vi "Example1.vi"() -> ()   [LabVIEW 2019]
uses:
  API/KafkaConsumerEvent.ctl
panel:
  out "size(s)":i32
  out "Events":T1[](array[typedef])
  in  "Topic":string="qamData"
  in  "Partition":i32
  in  "Kafka Broker":string="getafix.ni.corp.natinst.com:9092"
  in  "error in (no error)":errorcluster
  out "error out":errorcluster
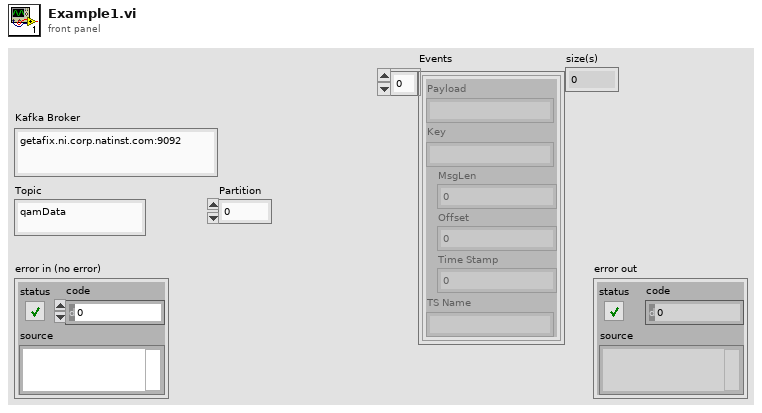
[diagram p1: front panel]
types:
  T1 = typedef "KafkaConsumerEvent.ctl" = cluster{"Payload":string, "Key":string, "MsgLen":u64, "Offset":i64, "Time Stamp":i64, "TS Name":string}
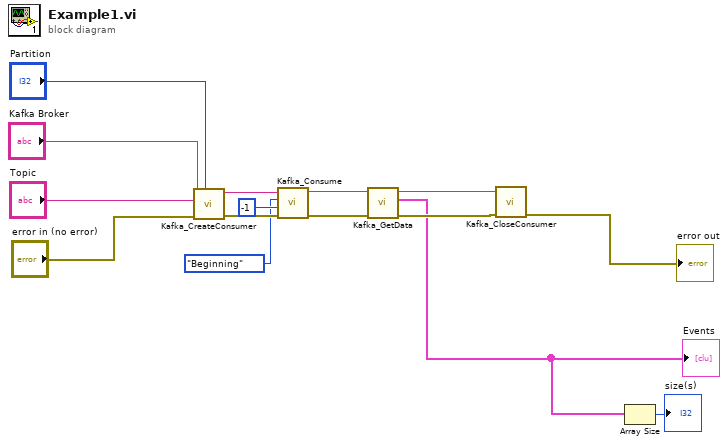
[diagram p0: block diagram]
diagram:
  n1 = call "Kafka_CreateConsumer.vi"("Partition"="Partition", "error in (no error)"="error in (no error)", "Topic"="Topic", "Kafka Broker"="Kafka Broker") -> ("error out"=w10:errorcluster, "Consumer Handle"=w9:string)  [unwired: 6 in]
  n2 = call "Kafka_Consume.vi"("error in (no error)"=w10, "Max Events"=i64 -1, "Kafka Offset"=enum16{"Beginning", "End", "Offset"}."Beginning", "Consumer Handle"=w9) -> ("error out"=w6:errorcluster, "Consumer Handle"=w4:string)  [unwired: 4 in, 2 out]
  n3 = call "Kafka_GetData.vi"("error in (no error)"=w6, "Consumer Handle"=w4) -> ("error out"=w5:errorcluster, "Events"=w2:T1[], "Consumer Handle"=w3:string)  [unwired: 7 in]
  "Events" <- w2
  n4 = call "Kafka_CloseConsumer.vi"("error in (no error)"=w5, "Consumer Handle"=w3) -> ("error out"=→"error out":errorcluster)  [unwired: 8 in, 1 out]
  n5 = Array Size(array=w2) -> (size(s)=→"size(s)":i32)
